vi "Contour2Path.vi"(11 "Polys":T3[](array[typedef])) -> (3 "Path":T2)   [LabVIEW 2014]
uses:
  TypeDefs/Poly2DwSlope.ctl
  TypeDefs/Point2DwSlope.ctl
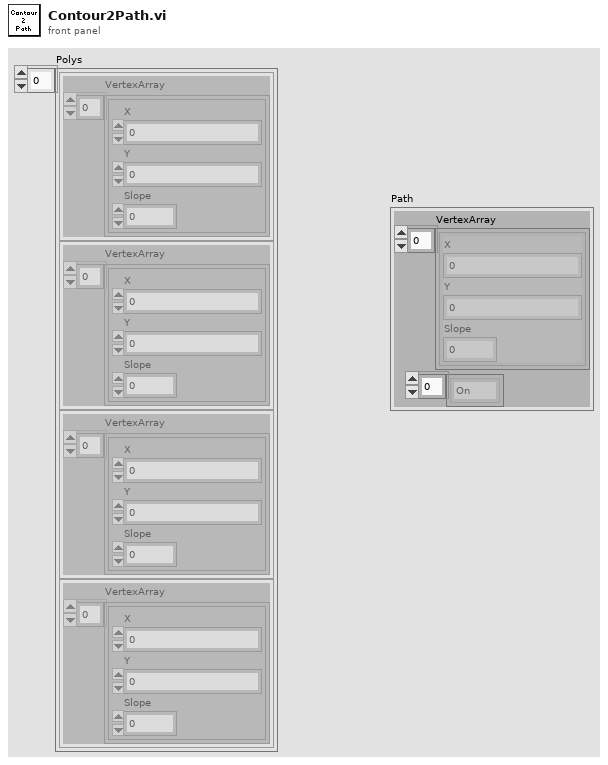
[diagram p1: front panel]
types:
  T1 = typedef "Point2DwSlope.ctl" = cluster{"X":sgl, "Y":sgl, "Slope":dbl}
  T2 = cluster{"VertexArray":T1[], enum16{"On", "Off"}[]}
  T3 = typedef "Poly2DwSlope.ctl" = cluster{"VertexArray":T1[]}
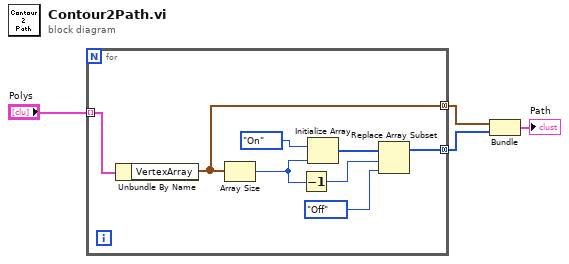
[diagram p0: block diagram]
diagram:
  n1 = for {
    tunnel: "Polys" -> [w12] mode=indexing
    tunnel: [w10] -> w3 mode=concatenating
    tunnel: [w8] -> w2 mode=concatenating
    n2 = Unbundle By Name(w12) -> ("VertexArray"=w10:T1[])
    n3 = Array Size(array=w10) -> (size(s)=w7:i32)
    n4 = Decrement(x=w7) -> (x-1=w6:i32)
    n5 = Initialize Array(enum16{"On", "Off"}."On", w7) -> (w9:enum16{"On", "Off"}[])
    n6 = Replace Array Subset(array=w9, new element=enum16{"On", "Off"}."Off" ("new element/subarray"), index=w6) -> (w8:enum16{"On", "Off"}[])
  }
  n7 = Bundle("VertexArray"=w3, w2) -> (→"Path":T2)  [unwired: 1 in]
